vi "Close.vi"(8 "error in (no error)":errorcluster, 11 "Pump in":T1) -> (0 "error out":errorcluster)   [LabVIEW 2017, in "Pump Controller.lvlib"]
uses:
  Pump Controller.lvlib
  Controls/Pump.ctl
  <instrlib>/Roboteq Controller KBL1xxx/Public/Controls/Controller.ctl
  <instrlib>/Roboteq Controller KBL1xxx/Roboteq Controller KBL1xxx.lvlib
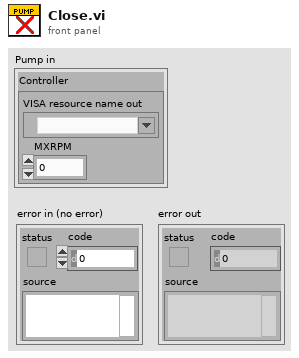
[diagram p1: front panel]
types:
  T1 = typedef "Pump Controller.lvlib/Pump.ctl" = cluster{"Controller":T2}
  T2 = typedef "Roboteq Controller KBL1xxx.lvlib/Controller.ctl" = cluster{"VISA resource name out":refnum<visa-resource-name>, "MXRPM":u16}
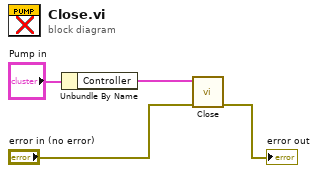
[diagram p0: block diagram]
diagram:
  n1 = Unbundle By Name("Pump in") -> ("Controller"=w3:T2)
  n2 = call <instrlib>:"Close.vi"("error in (no error)"="error in (no error)", "Controller in"=w3) -> ("error out"=→"error out":errorcluster)  [unwired: 9 in]
